vi "Scripts.vi"() -> ()   [LabVIEW 2018]
uses:
  InstrumentStatusLib/com.insstat.lvlib
panel:
  out "?":string
  out "?":string
  out "?":string
  out "?":bool
  out "?":string
  out "?":bool
  out "?":bool
  out "?":string
  out "?":bool
  out "?":bool
  out "?":string
  out "?":bool
  out "?":bool
  out "?":string
  out "?":bool
  out "?":string
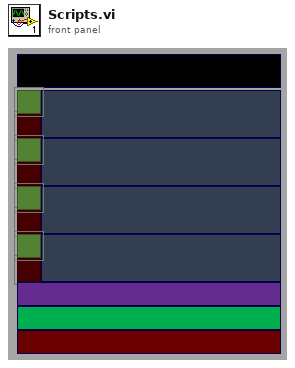
[diagram p1: front panel]
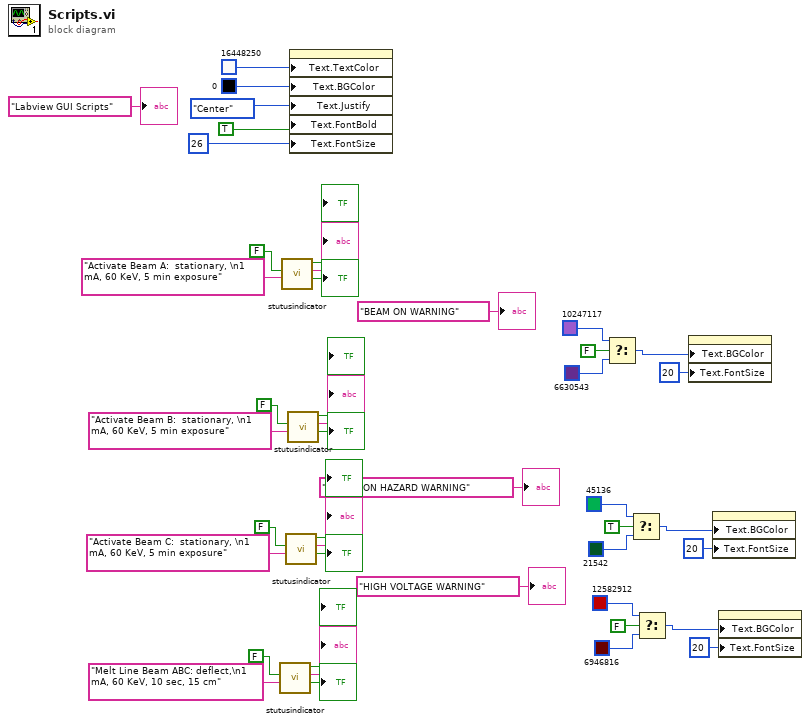
[diagram p0: block diagram]
diagram:
  n1 = call "stutusindicator.vi"("String"="Melt Line Beam ABC: deflect,\n1 mA, 60 KeV, 10 sec, 15 cm", "Boolean"=FALSE) -> (1:→"?":bool, 2:→"?":string, 3:→"?":bool)  [unwired: 7 in]
  n2 = call "stutusindicator.vi"("String"="Activate Beam A:  stationary, \n1 mA, 60 KeV, 5 min exposure", "Boolean"=FALSE) -> (1:→"?":bool, 2:→"?":string, 3:→"?":bool)  [unwired: 7 in]
  n3 = call "stutusindicator.vi"("String"="Activate Beam C:  stationary, \n1 mA, 60 KeV, 5 min exposure", "Boolean"=FALSE) -> (1:→"?":bool, 2:→"?":string, 3:→"?":bool)  [unwired: 7 in]
  n4 = call "stutusindicator.vi"("String"="Activate Beam B:  stationary, \n1 mA, 60 KeV, 5 min exposure", "Boolean"=FALSE) -> (1:→"?":bool, 2:→"?":string, 3:→"?":bool)  [unwired: 7 in]
  n5 = property class="Str"("Text.TextColor"=u32 16448250, "Text.BGColor"=u32 0, "Text.Justify"=enum16{"Left", "Center", "Right"}."Center" ("Text.Justification"), "Text.FontBold"=TRUE ("Text.Font:Bold"), "Text.FontSize"=u32 26 ("Text.Font:Size")) -> ()  [unwired: 2 in, 2 out]
  n6 = Select(t=u32 10247117, s=FALSE, f=u32 6630543) -> (s? t:f=w14:u32)
  n7 = Select(t=u32 45136, s=TRUE, f=u32 21542) -> (s? t:f=w8:u32)
  n8 = Select(t=u32 12582912, s=FALSE, f=u32 6946816) -> (s? t:f=w2:u32)
  n9 = property class="Str"("Text.BGColor"=w14, "Text.FontSize"=u32 20 ("Text.Font:Size")) -> ()  [unwired: 2 in, 2 out]
  n10 = property class="Str"("Text.BGColor"=w8, "Text.FontSize"=u32 20 ("Text.Font:Size")) -> ()  [unwired: 2 in, 2 out]
  n11 = property class="Str"("Text.BGColor"=w2, "Text.FontSize"=u32 20 ("Text.Font:Size")) -> ()  [unwired: 2 in, 2 out]
  "?" <- "Labview GUI Scripts" ("String")
  "?" <- "BEAM ON WARNING"
  "?" <- "RADIATION HAZARD WARNING"
  "?" <- "HIGH VOLTAGE WARNING"
